vi "Read.vi"(7 "timeout in ms (-1)":i32=-1, 8 "subchannel (0)":i32, 9 "ack id (0)":u32, 10 "channel":T1) -> (0 "last element?":bool, 1 "remaining":i32, 2 "element":T2, 3 "element valid?":bool, 5 "timed out?":bool)   [LabVIEW 2019, in "MessengerM.lvlib"]
doc: "Waits to read an element from a Messenger channel."
uses:
  <resource>/Channels/MessengerM/MessengerM.lvlib
  <resource>/Channels/MessengerM/))Channel.ctl
  <resource>/Channels/MessengerM/Element.ctl
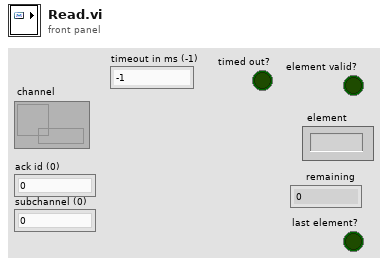
[diagram p1: front panel]
types:
  T1 = typedef "MessengerM.lvlib/))Channel.ctl" = refnum<queue>
  T2 = typedef "MessengerM.lvlib/Element.ctl" = string
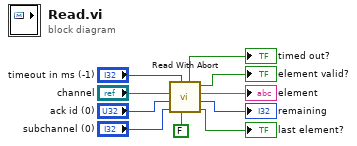
[diagram p0: block diagram]
diagram:
  n1 = call <resource>:"Read With Abort.vi"("abort (F)"=FALSE, "timeout in ms (-1)"="timeout in ms (-1)", "subchannel (0)"="subchannel (0)", "ack id (0)"="ack id (0)", "channel"="channel") -> ("last element?"=→"last element?":bool, "remaining"=→"remaining":i32, "element"=→"element":T2, "element valid?"=→"element valid?":bool, "timed out?"=→"timed out?":bool)  [unwired: 1 in, 1 out]
